vi "viewer test.vi"() -> ()   [LabVIEW 2015]
uses:
  <vilib>/ActorFramework/Actor/Actor.lvclass
  User Interface/Viewer/Viewer.lvclass
  Resources/GLOBAL/GLOBAL Time-critical.vi
  <vilib>/ActorFramework/Stop Msg/Stop Msg.lvclass
  Resources/C Libraries/histogram/histogram.dll
panel:
  out "x-y":u32
  out "Histogram":cluster{i32[], "Histogram":u64[]}(graph)
  in  "Boolean":bool
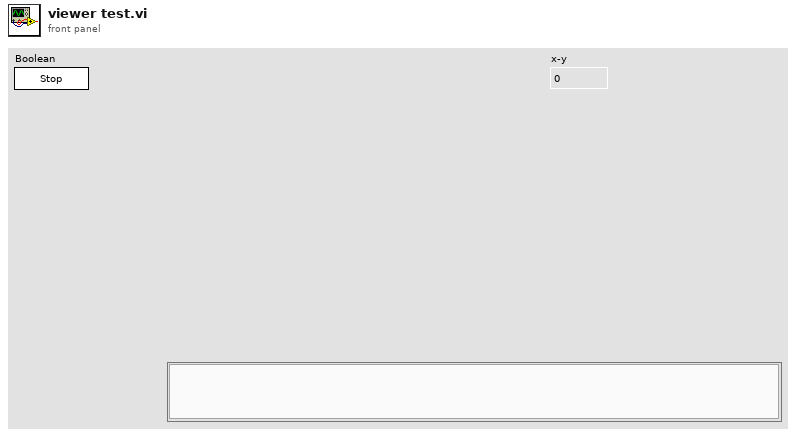
[diagram p1: front panel]
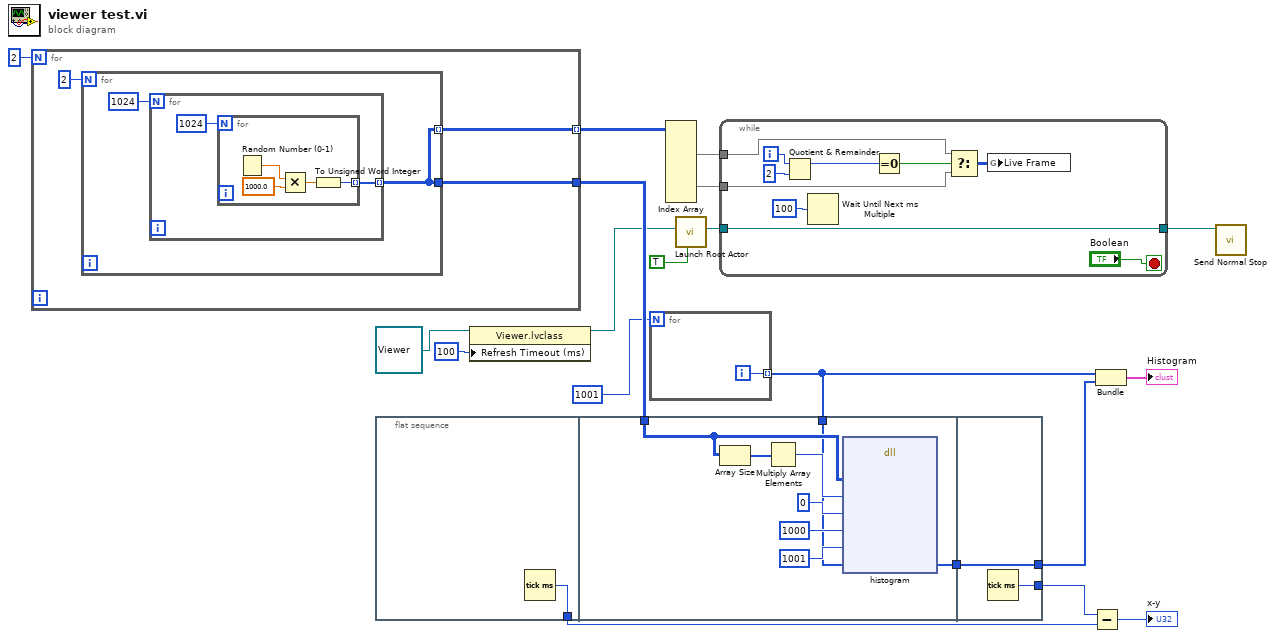
[diagram p0: block diagram]
diagram:
  n1 = for {
    N: 2 -> [_]
    tunnel: [w22] -> w18 mode=indexing
    tunnel: [w20] -> w17
    n2 = for {
      N: 2 -> [_]
      tunnel: [w23] -> w22 mode=indexing
      tunnel: [w23] -> w20
      n3 = for {
        N: 1024 -> [_]
        tunnel: [w25] -> w23 mode=indexing
        n4 = for {
          N: 1024 -> [_]
          tunnel: [w27] -> w25 mode=indexing
          n5 = Random Number (0-1)() -> (number: 0 to 1=w30:dbl)
          n6 = Multiply(x=w30, y=1000.0) -> (x*y=w28:dbl)
          n7 = To Unsigned Word Integer(number=w28) -> (unsigned 16bit integer=w27:u16)
        }
      }
    }
  }
  n8 = flat-sequence {
    tunnel: [w31] -> w15
    tunnel: w17 -> [w38]
    tunnel: [w34] -> w5
    tunnel: w1 -> [w32]
    tunnel: [w41] -> w16
    tunnel: w5 -> [w40]
    tunnel: [w40] -> w4
    frame #0 {
      n9 = Tick Count (ms)() -> (millisecond timer value=w31:u32)
    }
    frame #1 {
      n10 = Array Size(array=w38) -> (size(s)=w39:i32[])
      n11 = Multiply Array Elements(1:w39) -> (0:w37:i32)
      n12 = dll-call lib="C:/LV/Flash Gordon v0.5.6/Resources/C Libraries/histogram/histogram.dll" fn="histogram"("Frame"=w38, "Size"=w37, "Hist Min"=u16 0, "Hist Max"=u16 1000, "Bins"=u16 1001, "Histogram"=w32) -> ("Histogram"=w34:u64[])  [unwired: 9 in, 2 out]
    }
    frame #2 {
      n13 = Tick Count (ms)() -> (millisecond timer value=w41:u32)
    }
  }
  n14 = property class="Viewer.lvclass"(reference=refnum<class "Viewer.lvclass"> refnum ("Viewer.lvlib:Viewer.lvclass"), "Refresh Timeout (ms)"=100) -> (reference out=w11:refnum<class "Viewer.lvclass">)  [unwired: 1 in, 1 out]
  n15 = for {
    N: 1001 -> [_]
    tunnel: [w42] -> w1 mode=indexing
    i -> [w42]
  }
  n16 = Index Array(array=w18) -> (element #1=w8:u16[][][], element #2=w7:u16[][][])  [unwired: 8 in]
  n17 = call <vilib>:"Launch Root Actor.vi"("Open Actor Core front panel? (F)"=TRUE, "Actor"=w11) -> ("Actor's Enqueuer"=w9:refnum<class "Message Enqueuer.lvclass">)  [unwired: 8 in, 1 out]
  n18 = while {
    tunnel: w9 -> [w43]
    tunnel: w8 -> [w47]
    tunnel: w7 -> [w46]
    tunnel: [w43] -> w6
    i -> [w51]
    stop <- "Boolean" stop-if-true
    n19 = Quotient & Remainder(x=w51, y=2) -> (x-y*floor(x/y)=w49:i32)  [unwired: 1 out]
    n20 = Wait Until Next ms Multiple(millisecond multiple=u32 100) -> ()  [unwired: 1 out]
    n21 = Equal To 0?(x=w49) -> (x = 0?=w48:bool)
    n22 = Select(t=w47, s=w48, f=w46) -> (s? t:f=w45:u16[][][])
    n23 = global write "GLOBAL Time-critical.vi" "Live Frame"(w45) -> ()
  }
  n24 = Subtract(x=w16, y=w15) -> (x-y=→"x-y":u32)
  n25 = Bundle(w1, "Histogram"=w4) -> (→"Histogram":cluster{i32[], "Histogram":u64[]})  [unwired: 1 in]
  n26 = call <vilib>:"Send Normal Stop.vi"("Message Enqueuer"=w6) -> ()  [unwired: 10 in, 1 out]
